vi "powersweep.vi"() -> ()   [LabVIEW 2011]
panel:
  out "Numeric":i32
  out "Power (W)":dbl
  in  "Store file":path
  in  "Stop Button":bool
  out "current Q":i32
  out "Kinetic Series length":i32 min=0 step=1
  in  "Acquisition time [s]":dbl
  in  "Wavelength (nm)":dbl=350.0 min=350.0 max=1100.0 format="%#.1f"
  in  "step Q":i32 min=0 step=1
  in  "end Q":i32 min=0 step=1
  in  "start Q":i32 min=0 step=1
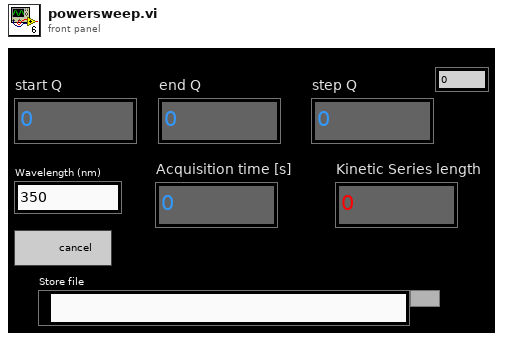
[diagram p1: front panel]
types:
  T1 = enum16{"open", "replace", "create", "open or create", "replace or create", "replace or create with confirmation"}
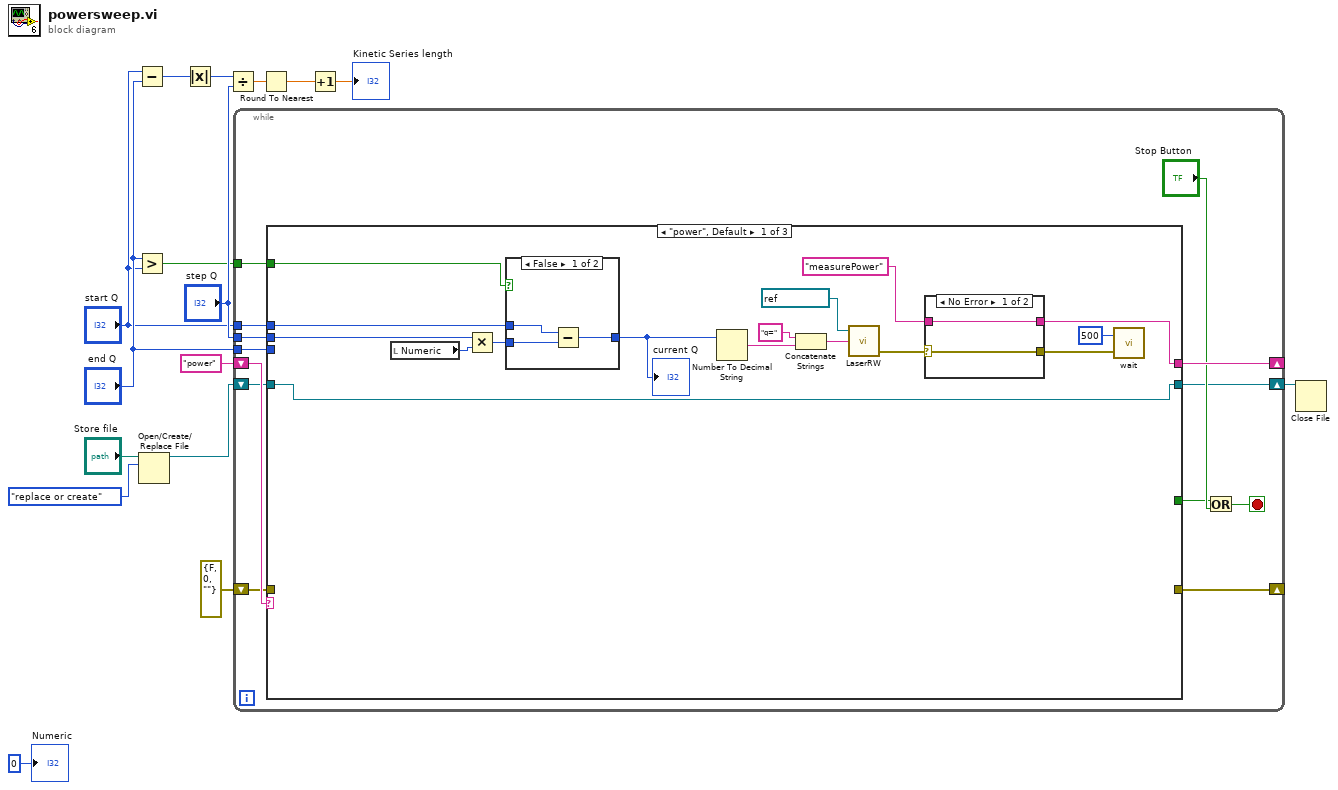
[diagram p0: block diagram]
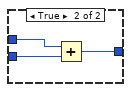
[diagram p2: hidden frame]
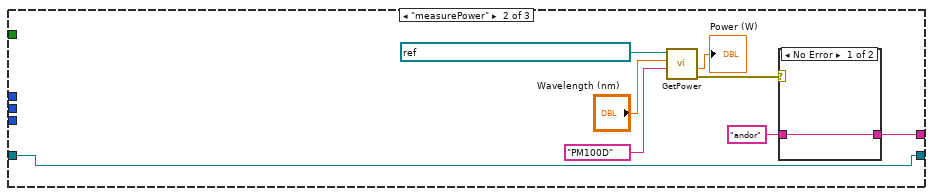
[diagram p4: hidden frame]
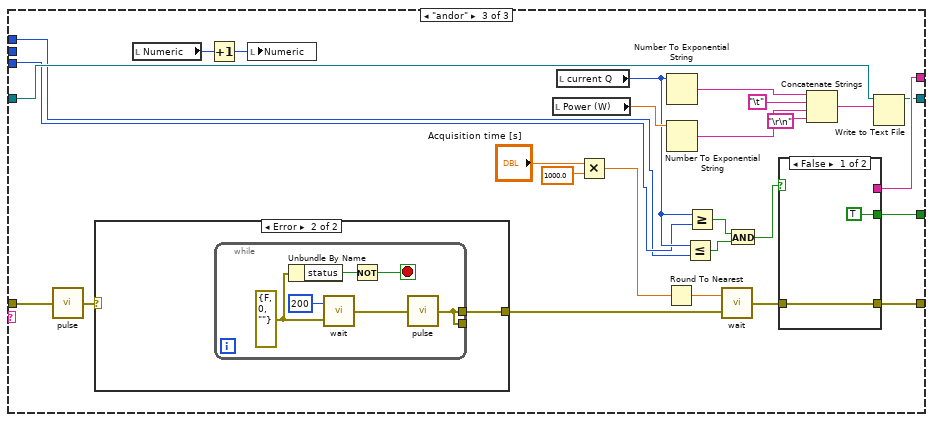
[diagram p6: hidden frame]
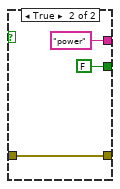
[diagram p7: hidden frame]
diagram:
  n1 = Subtract(x="start Q", y="end Q") -> (x-y=w15:i32)
  n2 = Greater?(x="end Q", y="start Q") -> (0:w1:bool)
  n3 = Open/Create/Replace File(file path (use dialog)="Store file", operation (0:open)=T1."replace or create") -> (refnum out=w10:refnum<file>)  [unwired: 4 in, 2 out]
  n4 = Absolute Value(x=w15) -> (abs(x)=w7:i32)
  n5 = Divide(x=w7, y="step Q") -> (x/y=w9:dbl)
  n6 = while {
    tunnel: "start Q" -> [w28]
    tunnel: "step Q" -> [w27]
    shift-right: [w26] -> _
    shift-left: "power" -> [w29]
    shift-right: [w24] -> _
    shift-left: errorcluster {"status"=FALSE, "code"=0, "source"=""} ("error in (no error)") -> [w25]
    tunnel: "end Q" -> [w23]
    shift-right: [w18] -> w8
    shift-left: w10 -> [w19]
    tunnel: w1 -> [w17]
    stop <- w20 stop-if-true
    n7 = case shown="\"power\", Default" w29 {
      tunnel: w28 -> [w45 _ w66]
      tunnel: w27 -> [w44 _ _]
      tunnel: [w43 w58 w85] -> w26
      tunnel: w25 -> [_ _ w92]
      tunnel: [_ _ w82] -> w24
      tunnel: w23 -> [_ _ w67]
      tunnel: [_ _ w84] -> w21
      tunnel: w19 -> [w42 w56 w75]
      tunnel: [w42 w56 w74] -> w18
      tunnel: w17 -> [w30 _ _]
      frame "power", Default {
        n8 = local read "Numeric"() -> (w31:i32)
        n9 = Multiply(x=w44, y=w31) -> (x*y=w39:i32)
        n10 = case shown="False" w30 {
          tunnel: w45 -> [w47 w51]
          tunnel: w39 -> [w48 w50]
          tunnel: [w46 w49] -> w38
          frame False {
            n11 = Subtract(x=w47, y=w48) -> (x-y=w46:i32)
          }
          frame True {
            n12 = Add(x=w51, y=w50) -> (x+y=w49:i32)
          }
        }
        "current Q" <- w38
        n13 = Number To Decimal String(number=w38) -> (decimal integer string=w37:string)  [unwired: 1 in]
        n14 = Concatenate Strings("q=" ("string"), w37) -> (w36:string)
        n15 = call "LaserRW.vi"("buffer à écrire"=w36, "Nom de ressource VISA"=refnum<visa-resource-name> "COM19") -> ("error out"=w35:errorcluster)  [unwired: 1 in, 2 out]
        n16 = case shown="No Error" w35 {
          selector: w35 -> [w52 w54]
          tunnel: "measurePower" -> [w53 w55]
          tunnel: [w53 w55] -> w43
          tunnel: [w52 w54] -> w33
          frame No Error {
          }
          frame Error {
          }
        }
        n17 = call "wait.vi"("error in (no error)"=w33, "wait time"=500) -> ()  [unwired: 1 out]
      }
      frame "measurePower" {
        n18 = call "GetPower.vi"("Measeaurement mode"="PM100D", "Wavelength (nm)"="Wavelength (nm)", "Input Device"=refnum<visa-resource-name> "USB0::0x1313::0x8072::P2007928::INSTR") -> ("error out"=w60:errorcluster, "Power (W)"=→"Power (W)":dbl)  [unwired: 1 in, 2 out]
        n19 = case shown="No Error" w60 {
          tunnel: "andor" -> [w64 w65]
          tunnel: [w64 w65] -> w58
          frame No Error {
          }
          frame Error {
          }
        }
      }
      frame "andor" {
        n20 = call "pulse.vi"("error in"=w92) -> ("error out"=w87:errorcluster)
        n21 = case shown="Error" w87 {
          selector: w87 -> [w98 _]
          tunnel: [w98 w99] -> w86
          frame No Error {
          }
          frame Error {
            n22 = while {
              tunnel: [w100] -> _
              tunnel: [w100] -> w99
              stop <- w101 stop-if-true
              w103 = errorcluster {"status"=FALSE, "code"=0, "source"=""} ("error in")
              n23 = Unbundle By Name(w103) -> ("status"=w102:bool)
              n24 = call "wait.vi"("error in (no error)"=w103, "wait time"=200) -> ("error in (no error) 2"=w104:errorcluster)
              n25 = Not(x=w102) -> (.not. x?=w101:bool)
              n26 = call "pulse.vi"("error in"=w104) -> ("error out"=w100:errorcluster)
            }
          }
        }
        n27 = local read "Numeric"() -> (w73:i32)
        n28 = Increment(x=w73) -> (x+1=w72:i32)
        n29 = local write "Numeric"(w72) -> ()
        n30 = local read "Power (W)"() -> (w78:dbl)
        n31 = local read "current Q"() -> (w71:i32)
        n32 = Multiply(x="Acquisition time [s]", y=1000.0) -> (x*y=w89:dbl)
        n33 = Round To Nearest(number=w89) -> (nearest integer value=w88:dbl)
        n34 = Number To Exponential String(number=w71) -> (E-format string=w80:string)  [unwired: 3 in]
        n35 = Number To Exponential String(number=w78) -> (E-format string=w77:string)  [unwired: 3 in]
        n36 = Less Or Equal?(x=w71, y=w66) -> (x <= y?=w70:bool)
        n37 = Greater Or Equal?(x=w71, y=w67) -> (x >= y?=w69:bool)
        n38 = call "wait.vi"("error in (no error)"=w86, "wait time"=w88) -> ("error in (no error) 2"=w83:errorcluster)
        n39 = And(x=w69, y=w70) -> (x .and. y?=w68:bool)
        n40 = case shown="False" w68 {
          tunnel: [_ "power"] -> w85
          tunnel: [TRUE FALSE] -> w84
          tunnel: w83 -> [w93 w95]
          tunnel: [w93 w95] -> w82
          frame False {
          }
          frame True {
          }
        }
        n41 = Concatenate Strings(w80, "\t", w77, "\r\n") -> (w79:string)
        n42 = Write to Text File(file (use dialog)=w75, text=w79) -> (refnum out=w74:refnum<file>)  [unwired: 2 in, 2 out]
      }
    }
    n43 = Or(x=w21, y="Stop Button") -> (x .or. y?=w20:bool)
  }
  n44 = Round To Nearest(number=w9) -> (nearest integer value=w6:dbl)
  n45 = Increment(x=w6) -> (x+1=→"Kinetic Series length":dbl)
  n46 = Close File(refnum=w8) -> ()  [unwired: 1 in, 2 out]
  "Numeric" <- 0 ("Numeric")
